vi "Word_Get_Properties.vi"(0 "report in":refnum<class "NI_report.lvclass">, 11 "error in (no error)":errorcluster) -> (4 "report out":refnum<class "NI_report.lvclass">, 6 "tables count":i32, 8 "shapes count":i32, 10 "document count":i32, 14 "character count":i32, 15 "error out":errorcluster)   [LabVIEW 2020, in "NI_Word.lvclass"]
doc: "Gets the number of worksheets in the active workbook."
uses:
  <vilib>/Utility/NIReport.llb/Word/NI_Word.lvclass
  <vilib>/Utility/NIReport.llb/NI_report.lvclass
  C:/Program Files (x86)/National Instruments/LabVIEW 2020/vi.lib/Utility/NIReport.llb/NI_report.lvclass
  <vilib>/Utility/NIReport.llb/Word/NI_Word.lvclass/NI_Word.ctl
  <vilib>/Utility/NIReport.llb/NI_ReportGenerationCore.lvlib
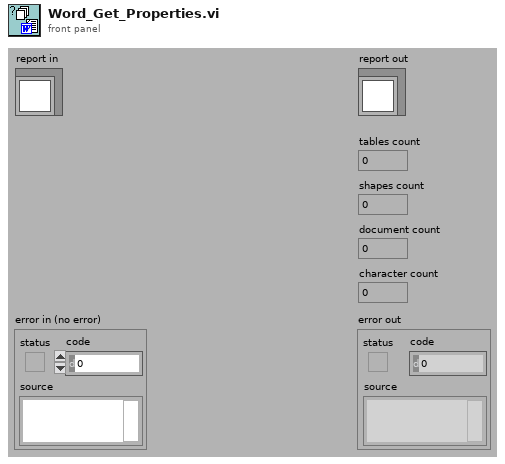
[diagram p1: front panel]
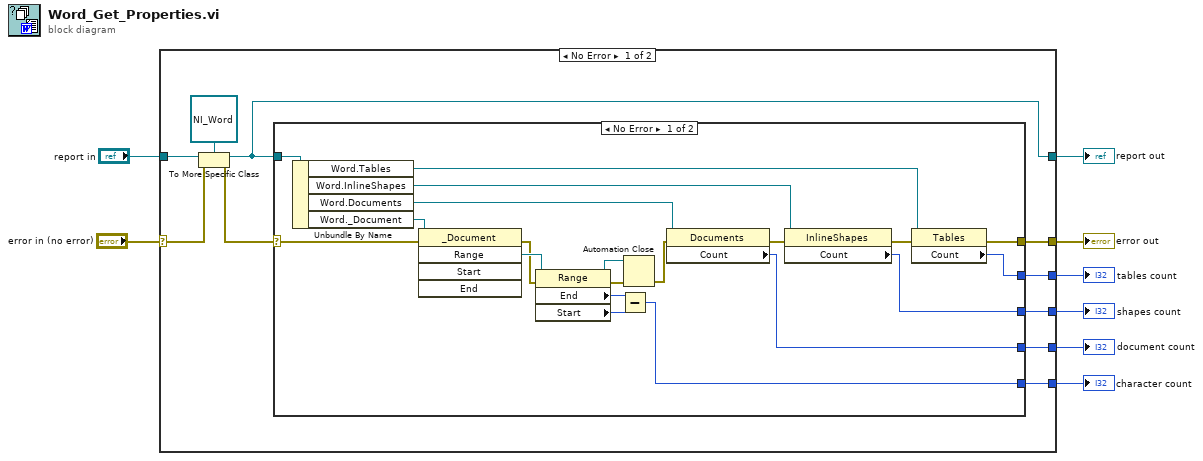
[diagram p0: block diagram]
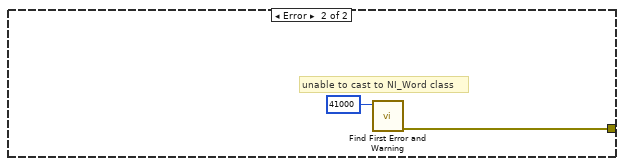
[diagram p2: hidden frame]
diagram:
  n1 = case shown="No Error" "error in (no error)" {
    selector: "error in (no error)" -> [w10 w42]
    tunnel: [w18 w42] -> w7
    tunnel: [w12 w41] -> w5
    tunnel: "report in" -> [w13 w41]
    tunnel: [w17 _] -> w4
    tunnel: [w16 _] -> w3
    tunnel: [w15 _] -> w2
    tunnel: [w9 _] -> w1
    frame No Error {
      n2 = To More Specific Class(target class=refnum<class "NI_Word.lvclass"> refnum ("report in"), reference=w13, error in=w10) -> (specific class reference=w12:refnum<class "NI_Word.lvclass">, error out=w11:errorcluster)
      n3 = case shown="No Error" w11 {
        selector: w11 -> [w28 _]
        tunnel: [w33 w39] -> w18
        tunnel: [w32 _] -> w17
        tunnel: [w31 _] -> w16
        tunnel: [w30 _] -> w15
        tunnel: w12 -> [w29 _]
        tunnel: [w19 _] -> w9
        frame No Error {
          n4 = Unbundle By Name(w29) -> ("Word.Tables"=w38:refnum<k7>, "Word.InlineShapes"=w35:refnum<k7>, "Word.Documents"=w36:refnum<k7>, "Word._Document"=w27:refnum<k7>)
          n5 = invoke class="_Document" method="Range"(reference=w27, error in=w28) -> (error out=w21:errorcluster, "Range"=w22:refnum<k7>)  [unwired: 3 in, 3 out]
          n6 = property class="Range"(reference=w22, error in=w21) -> (reference out=w26:refnum<k7>, error out=w25:errorcluster, "End"=w23:i32, "Start"=w24:i32)
          n7 = Subtract(x=w23, y=w24) -> (x-y=w19:i32)
          n8 = Automation Close(3:w25, 5:w26) -> (0:w20:errorcluster)
          n9 = property class="Documents"(reference=w36, error in=w20) -> (error out=w37:errorcluster, "Count"=w30:i32)  [unwired: 1 out]
          n10 = property class="InlineShapes"(reference=w35, error in=w37) -> (error out=w34:errorcluster, "Count"=w31:i32)  [unwired: 1 out]
          n11 = property class="Tables"(reference=w38, error in=w34) -> (error out=w33:errorcluster, "Count"=w32:i32)  [unwired: 1 out]
        }
        frame Error {
          # "unable to cast to NI_Word class"
          n12 = call <vilib>:"Find First Error and Warning.vi"("error code"=41000) -> ("error out"=w39:errorcluster)  [unwired: 2 in, 4 out]
        }
      }
    }
    frame Error {
    }
  }
  "error out" <- w7
  "report out" <- w5
  "tables count" <- w4
  "shapes count" <- w3
  "document count" <- w2
  "character count" <- w1
